vi "Julabo Test Program.vi"() -> ()   [LabVIEW 2018, in "Julabo Type FP-50 TCU.lvlib"]
uses:
  Julabo Type FP-50 TCU.lvlib
  Julabo FP-50 Settings.ctl
panel:
  out "Pumpstage (out)":u8
  out "Temp Out":dbl
  in  "Internal?":bool
  out "Running":bool
  out "Connection Error":bool
  in  "stop":bool
  in  "Temp":dbl
  in  "Run":bool
  out "error out":errorcluster
  in  "error in (no error)":errorcluster
  out "Julabo Settings":T1={"VISA resource name"="", "Simulated?"=FALSE, "Pump Power"=2} {"Pump Power" min=0 max=8 step=1}
  in  "Julabo Settings":T1={"VISA resource name"="", "Simulated?"=FALSE, "Pump Power"=2} {"Pump Power" min=0 max=8 step=1}
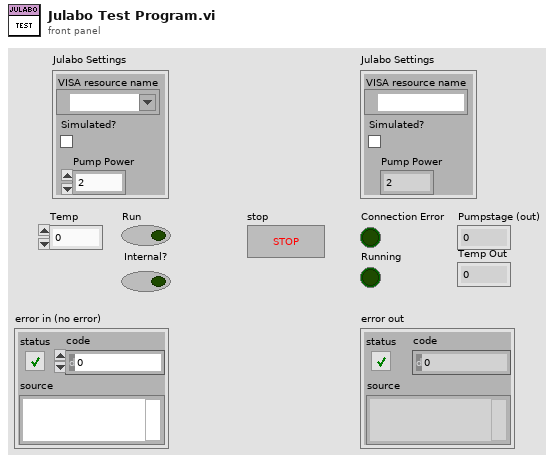
[diagram p1: front panel]
types:
  T1 = typedef "Julabo Type FP-50 TCU.lvlib/Julabo FP-50 Settings.ctl" = cluster{"VISA resource name":refnum<visa-resource-name>, "Simulated?":bool, "Pump Power":i32}
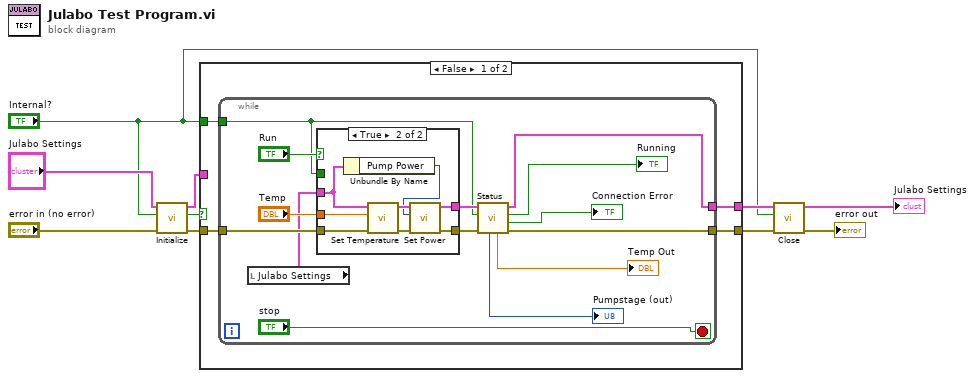
[diagram p0: block diagram]
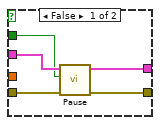
[diagram p2: hidden frame]
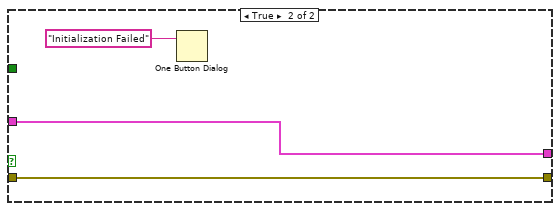
[diagram p3: hidden frame]
diagram:
  n1 = call "Initialize.vi"("error in (no error)"="error in (no error)", "Internal?"="Internal?", "Julabo FP-50 Settings"="Julabo Settings") -> ("error out"=w3:errorcluster, "Connection Error"=w2:bool, "Julabo FP-50 Settings"=w4:T1)  [unwired: 6 in]
  n2 = case shown="False" w2 {
    tunnel: [w14 w43] -> w8
    tunnel: [w13 w42] -> w6
    tunnel: w4 -> [_ w43]
    tunnel: w3 -> [w12 w42]
    tunnel: "Internal?" -> [w11 _]
    frame False {
      n3 = while {
        tunnel: [w28] -> w14
        tunnel: [w27] -> w13
        tunnel: w12 -> [w25]
        tunnel: w11 -> [w18]
        stop <- "stop" stop-if-true
        n4 = local read "Julabo Settings"() -> (w15:T1)
        n5 = case shown="True" "Run" {
          tunnel: w15 -> [w33 w35]
          tunnel: w25 -> [w32 w41]
          tunnel: [w31 w36] -> w24
          tunnel: [w30 w38] -> w23
          tunnel: "Temp" -> [_ w40]
          tunnel: w18 -> [w29 _]
          frame False {
            n6 = call "Pause.vi"("error in (no error)"=w32, "Internal?"=w29, "Julabo FP-50 Settings In"=w33) -> ("error out"=w31:errorcluster, "Julabo FP-50 Settings Out"=w30:T1)  [unwired: 7 in]
          }
          frame True {
            n7 = Unbundle By Name(w35) -> ("Pump Power"=w34:i32)
            n8 = call "Set Temperature.vi"("error in (no error)"=w41, "Setpoint"=w40, "Julabo Fp-50 Settings"=w35) -> ("error out"=w37:errorcluster, "Julabo FP-50 Settings"=w39:T1)  [unwired: 6 in, 1 out]
            n9 = call "Set Power.vi"("error in (no error)"=w37, "Power"=w34, "Julabo FP-50 Settings"=w39) -> ("error out"=w36:errorcluster, "Julabo FP-50 Settings"=w38:T1)  [unwired: 6 in, 1 out]
          }
        }
        n10 = call "Status.vi"("error in (no error)"=w24, "Internal?"=w18, "Julabo FP-50 Settings In"=w23) -> ("error out"=w27:errorcluster, "Connection Error"=→"Connection Error":bool, "Running"=→"Running":bool, "Julabo FP-50 Settings Out"=w28:T1, "Temp"=→"Temp Out":dbl, "Pumpstage (out)"=→"Pumpstage (out)":u8)  [unwired: 3 in]
      }
    }
    frame True {
      n11 = One Button Dialog(message="Initialization Failed") -> ()  [unwired: 1 in, 1 out]
    }
  }
  n12 = call "Close.vi"("error in (no error)"=w6, "Internal?"="Internal?", "Julabo Fp-50 Settings"=w8) -> ("error out"=→"error out":errorcluster, "Julabo FP-50 Settings"=→"Julabo Settings":T1)  [unwired: 7 in]
